vi "Test Move To Name.vi"() -> ()   [LabVIEW 2011]
uses:
  Config Manager Class/Type Definitions/Named Position.ctl
  Gantry Class.lvclass
panel:
  in  "Array":T1[](array[typedef])=[enum."module_chuck_0", enum."glue_reservoir_chuck", enum."tool_rack_pos_1_in", enum."home"]
  out "error out":errorcluster
  in  "Config Folder":path=path "C:/Users/Husker/Desktop/gantry/Config"
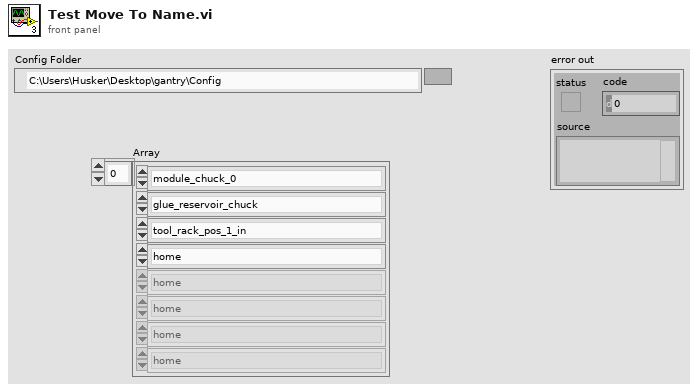
[diagram p1: front panel]
types:
  T1 = typedef "Named Position.ctl" = enum16{"home", "module_chuck_0", "module_chuck_1", "module_chuck_2", "module_chuck_3", "module_chuck_4", "glue_reservoir_chuck", "stamp_tool_chuck", "weight_tool_chuck", "needle_calibration", "needle_calibration_camera", "tool_rack_pos_0_in", "tool_rack_pos_0_out", "tool_rack_pos_1_in", "tool_rack_pos_1_out", "tool_rack_pos_2_in", "tool_rack_pos_2_out", "front_load_position", "grabber_start_pos", "between_chuck_0_and_1", "between_chuck_2_and_3"}
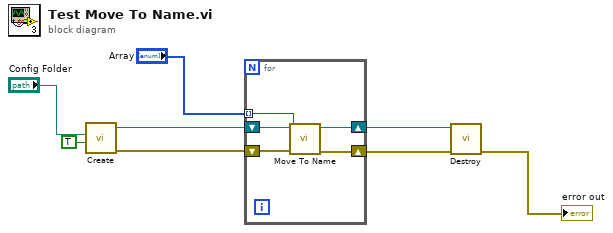
[diagram p0: block diagram]
diagram:
  n1 = call "Create.vi"("HOME?"=TRUE, "Config Folder"="Config Folder") -> ("error out"=w5:errorcluster, "Gantry out"=w6:refnum<class "Gantry Class.lvclass">)  [unwired: 8 in]
  n2 = for {
    tunnel: "Array" -> [w12] mode=indexing
    shift-right: [w10] -> w4
    shift-left: w6 -> [w13]
    shift-right: [w9] -> w3
    shift-left: w5 -> [w11]
    n3 = call-dynamic "Move To Name.vi"("error in"=w11, "Destination"=w12, "Gantry in"=w13) -> ("error out"=w9:errorcluster, "Gantry out"=w10:refnum<class "Gantry Class.lvclass">)  [unwired: 7 in]
  }
  n4 = call "Destroy.vi"("error in"=w3, "Gantry Class in"=w4) -> ("error out"=→"error out":errorcluster)  [unwired: 9 in]
